vi "Initialize Default.vi"(8 "error in (no error)":errorcluster, 11 "UDP Rx Transfer Configuration in":refnum<class "UDP Transfer Rx Configuration.lvclass">) -> (0 "error out":errorcluster, 3 "UDP Rx Transfer Configuration out":refnum<class "UDP Transfer Rx Configuration.lvclass">)   [LabVIEW 2017, in "UDP Transfer Rx Configuration.lvclass"]
uses:
  UDP Transfer Rx Configuration.lvclass
  UDP Transfer Rx Configuration.lvclass/UDP Transfer Rx Configuration.ctl
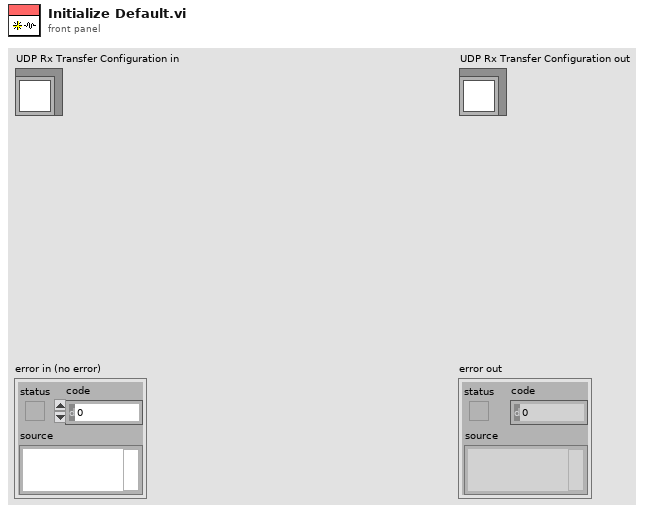
[diagram p1: front panel]
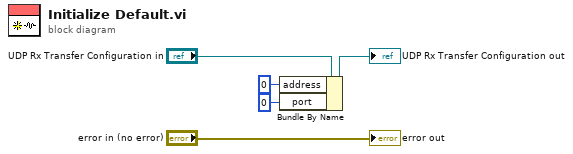
[diagram p0: block diagram]
diagram:
  n1 = Bundle By Name(cluster="UDP Rx Transfer Configuration in", "address"=u32 0 ("rx transfer settings.address"), "port"=u16 0 ("rx transfer settings.port")) -> (→"UDP Rx Transfer Configuration out":refnum<class "UDP Transfer Rx Configuration.lvclass">)
  "error out" <- "error in (no error)"
